vi "Get-active-clients.vi"(8 "error in (no error)":errorcluster, 11 "ModComm in":T2) -> (0 "error out":errorcluster, 2 "Active clients":T1(array[cluster]), 3 "ModComm out":T2)   [LabVIEW 2013, in "Server.lvlib" / "Server.lvclass"]
uses:
  Server.lvclass
  Object-reference.ctl
  Server.lvclass/Server.ctl
  Read Clients.vi
  Read Client IDs.vi
  Read Last contact.vi
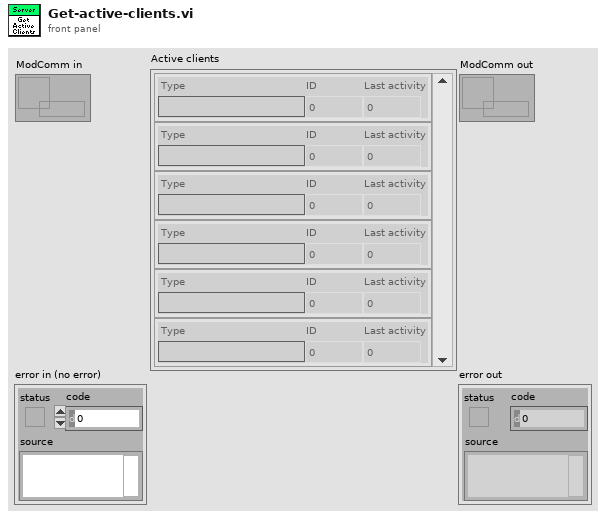
[diagram p1: front panel]
types:
  T1 = cluster{"Type":string, "ID":i32, "Last activity":i32}[]
  T2 = typedef "Server.lvlib/Server.lvclass/Object-reference.ctl" = refnum<data-value>
  T3 = cluster{"Type":string, "ID":i32, "Last activity":i32}
  T4 = typedef "Module-communication.lvlib/Server.lvclass/Supported-module-types.ctl" = enum16{"Server", "All", "BeamControl", "PowderDeposition", "StrategyParser", "CameraVision", "MaterialCharacterization", "StatusMonitor", "SLMSimulation", "LaserCharacterization"}
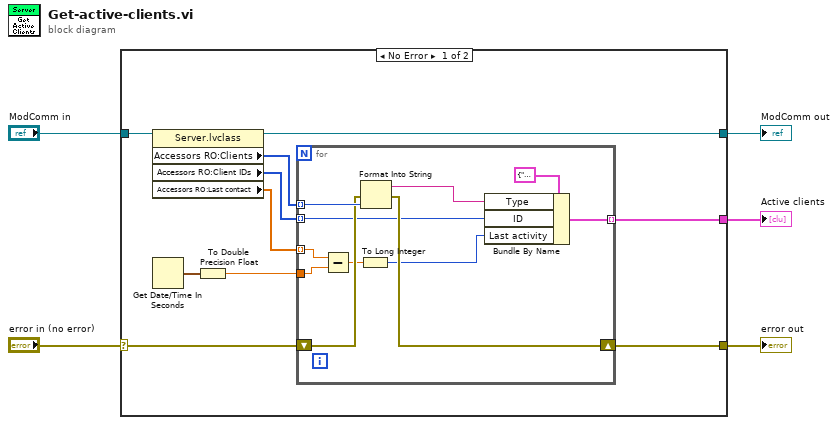
[diagram p0: block diagram]
diagram:
  n1 = case shown="No Error" "error in (no error)" {
    selector: "error in (no error)" -> [w9 w28]
    tunnel: [w6 w28] -> w4
    tunnel: [w7 w27] -> w2
    tunnel: "ModComm in" -> [w15 w27]
    tunnel: [w8 _] -> w1
    frame No Error {
      n2 = property class="Server.lvclass"(reference=w15) -> (reference out=w7:T2, "Accessors RO:Clients"=w13:T4[], "Accessors RO:Client IDs"=w12:i32[], "Accessors RO:Last contact"=w11:dbl[])  [unwired: 1 in, 1 out]
      n3 = Get Date/Time In Seconds() -> (seconds since 1Jan1904=w14:timestamp)
      n4 = To Double Precision Float(number=w14) -> (double precision float=w10:dbl)
      n5 = for {
        tunnel: w13 -> [w23] mode=indexing
        tunnel: w12 -> [w19] mode=indexing
        tunnel: w11 -> [w25] mode=indexing
        tunnel: w10 -> [w26]
        shift-right: [w21] -> w6
        shift-left: w9 -> [w22]
        tunnel: [w16] -> w8 mode=indexing
        n6 = Subtract(x=w25, y=w26) -> (x-y=w18:dbl)
        n7 = To Long Integer(number=w18) -> (32bit integer=w17:i32)
        n8 = Format Into String(error in=w22, w23) -> (resulting string=w20:string, error out=w21:errorcluster)  [unwired: 2 in]
        n9 = Bundle By Name(cluster=T3 {"Type"="", "ID"=0, "Last activity"=0} ("Client"), "Type"=w20, "ID"=w19, "Last activity"=w17) -> (w16:T3)
      }
    }
    frame Error {
    }
  }
  "error out" <- w4
  "ModComm out" <- w2
  "Active clients" <- w1
